vi "OPO_q_switch.vi"(3 "error in (no error)":errorcluster, 4 "display_message":bool, 5 "qindicator":refnum<vi>) -> (0 "error out":errorcluster, 2 "OK":bool)   [LabVIEW 2019]
doc: "This VI checks that OPO is still q switching. OK goes to True if it fails"
uses:
  Action spectra/Set wavelength.vi
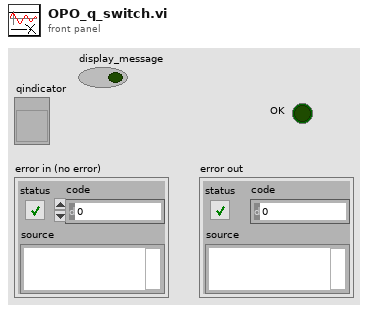
[diagram p1: front panel]
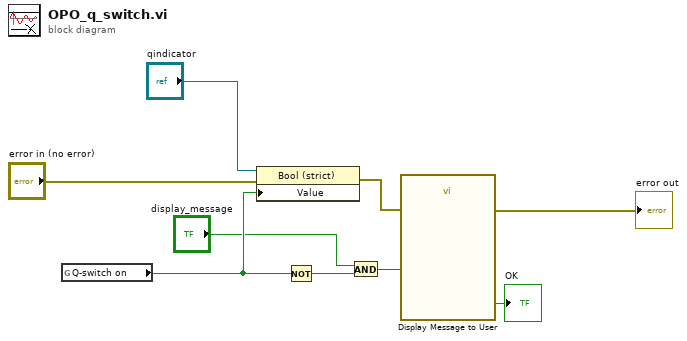
[diagram p0: block diagram]
diagram:
  n1 = global read "Set wavelength.vi" "Q-switch on"() -> (w6:bool)
  n2 = property on="Property Node" class="Bool (strict)"(reference="qindicator", error in="error in (no error)", "Value"=w6) -> (error out=w8:errorcluster)  [unwired: 1 out]
  n3 = Not(x=w6) -> (.not. x?=w7:bool)
  n4 = And(x="display_message", y=w7) -> (x .and. y?=w2:bool)
  n5 = call "Display Message to User"("error in (no error)"=w8, "Enable"=w2) -> ("error out"=→"error out":errorcluster, "OK"=→"OK":bool)  [unwired: 8 in]
